vi "Read Sim Image.vi"(8 "error in (no error)":errorcluster, 11 "Sim Camera Driver in":refnum<class "Sim Camera Driver.lvclass">) -> (0 "error out":errorcluster, 2 "Sim Image":path, 3 "Sim Camera Driver out":refnum<class "Sim Camera Driver.lvclass">)   [LabVIEW 2022 SP3, in "Sim Camera Driver.lvclass"]
uses:
  Sim Camera Driver.lvclass
  Sim Camera Driver.lvclass/Sim Camera Driver.ctl
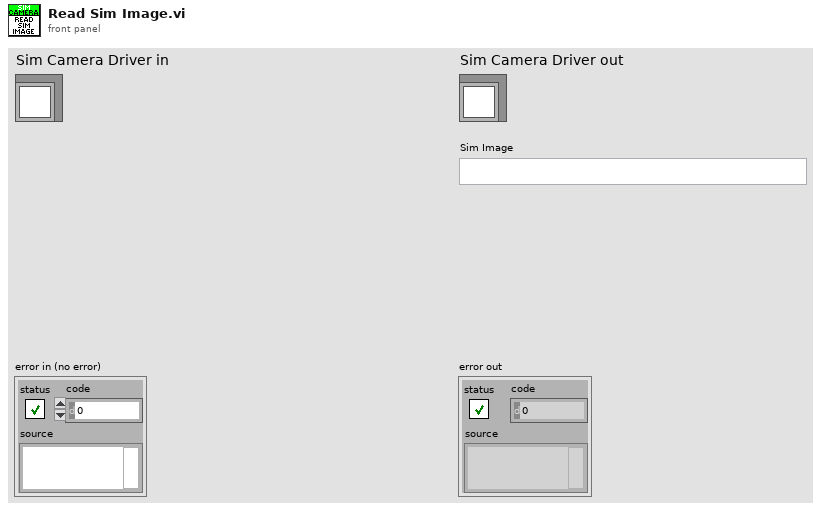
[diagram p1: front panel]
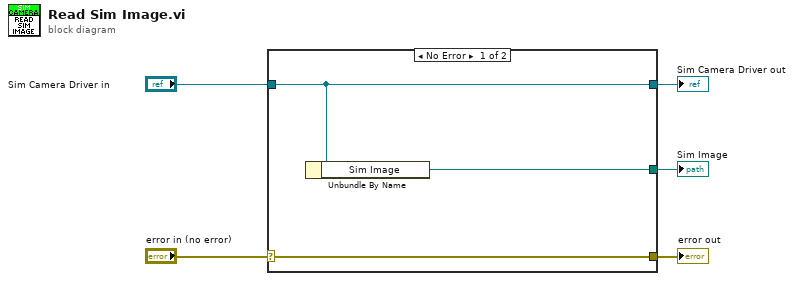
[diagram p0: block diagram]
diagram:
  n1 = case shown="No Error" "error in (no error)" {
    selector: "error in (no error)" -> [w8 w9]
    tunnel: [w8 w9] -> w4
    tunnel: [w7 w10] -> w2
    tunnel: "Sim Camera Driver in" -> [w7 w10]
    tunnel: [w6 _] -> w1
    frame No Error {
      n2 = Unbundle By Name(w7) -> ("Sim Image"=w6:path)
    }
    frame Error {
    }
  }
  "error out" <- w4
  "Sim Camera Driver out" <- w2
  "Sim Image" <- w1
